vi "Shooter Speed.vi"() -> ()   [LabVIEW 2013]
uses:
  Shooter Speed Global.vi
panel:
  in  "Battery Voltage":dbl(slide)=12.0 scale=12.0..13.0
  in  "Output at 13v":dbl(slide)=0.7 scale=0.7..0.9
  in  "Output at 12v":dbl(slide)=0.9 scale=0.7..0.9
  out "Motor Output":dbl(knob) scale=0.7..0.9
  # "Click          to run"
  # "Shooter Speed"
  # "Play around with these values to see if it works"
  # "In 2013, the game required us to shoot frisbees, which was done using a wheel. The system looked similar to this illustration (figure 1). \nWe wanted this wheel to spin at a constant rate, but this is difficult because different batteries will have different voltages. If set the motor to an output of 0.8 (with 1.0 as maximum), it will spin at a slower speed with a 12.0v battery than with a 13.0v battery.\nIn order to compensate for this, we used a linear function that would set the motor to a higher output for weaker batteries (figure 2). First, we found the optimal motor output for a battery with 12v, then found the optimal output for 13v. Using this data, we could In retrospect, using an encoder to directly measure the RPM would have been better, and we will probably do that if any upcoming games require a shooter wheel.\n\nYour task is to create this linear function. \nIf you have taken Algebra 1, you should be familiar with slope intercept form: y = mx + b. \nTo review on the math, finding the slope (m) of the function can be done with: (y2-y1) / (x2- x1)\nTo find the y-intercept (b), plug in any x (voltage) and its corresponding y (output), then solve for b.\n\nIf you haven't seen linear functions before, but still want to do this exercise, send me an email.\n(cjl2625@gmail.com)"
  # "figure 1"
  # "figure 2"
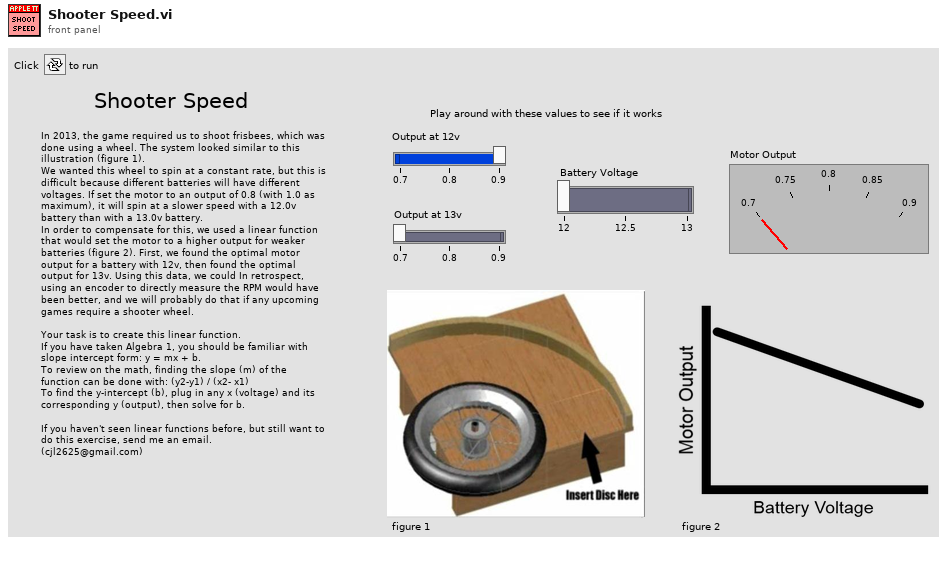
[diagram p1: front panel]
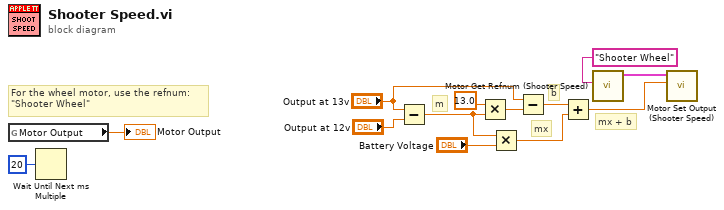
[diagram p0: block diagram]
diagram:
  # "mx + b"
  # "mx"
  # "b"
  # "m"
  # "For the wheel motor, use the refnum:\n\"Shooter Wheel\""
  n1 = global read "Shooter Speed Global.vi" "Motor Output"() -> (→"Motor Output":dbl)
  n2 = Wait Until Next ms Multiple(millisecond multiple=u32 20) -> ()  [unwired: 1 out]
  n3 = Subtract(x="Output at 13v", y="Output at 12v") -> (x-y=w6:dbl)
  n4 = Multiply(x=13.0, y=w6) -> (x*y=w9:dbl)
  n5 = Multiply(x=w6, y="Battery Voltage") -> (x*y=w4:dbl)
  n6 = Subtract(x="Output at 13v", y=w9) -> (x-y=w7:dbl)
  n7 = Add(x=w7, y=w4) -> (x+y=w1:dbl)
  n8 = call "Motor Get Refnum (Shooter Speed).vi"("refnum name"="Shooter Wheel") -> ("MotorControlDevRef"=w3:cluster{string, i32})  [unwired: 9 in, 1 out]
  n9 = call "Motor Set Output (Shooter Speed).vi"("Output"=w1, "MotorControlDevRef"=w3) -> ()  [unwired: 7 in, 3 out]
